vi "Write SC2250 TX Resource Name.vi"(8 "error in (no error)":errorcluster, 10 "SC2250 TX Resource Name":string, 11 "SG SC2250 Path in":refnum<class "SG SC2250 Path.lvclass">) -> (0 "error out":errorcluster, 3 "SG SC2250 Path out":refnum<class "SG SC2250 Path.lvclass">)   [LabVIEW 2023, in "RFFixtureCharact.RFPM.lvlib" / "SG SC2250 Path.lvclass"]
uses:
  SG SC2250 Path.lvclass
  SG SC2250 Path.lvclass/SG SC2250 Path.ctl
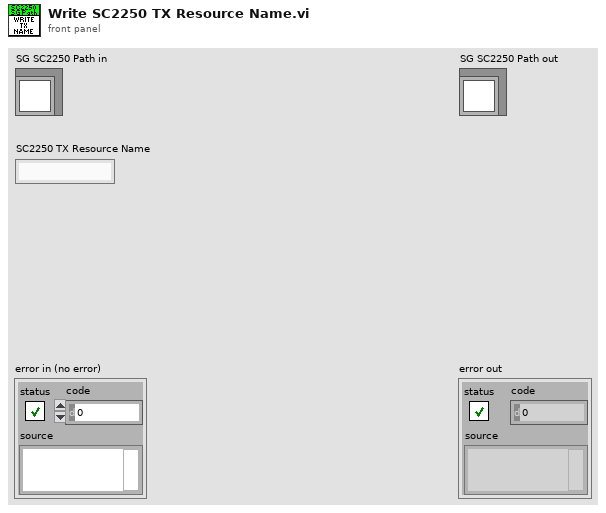
[diagram p1: front panel]
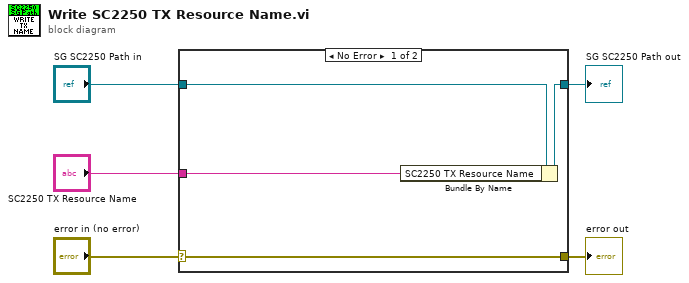
[diagram p0: block diagram]
diagram:
  n1 = case shown="No Error" "error in (no error)" {
    selector: "error in (no error)" -> [w9 w10]
    tunnel: [w9 w10] -> w4
    tunnel: [w7 w11] -> w2
    tunnel: "SG SC2250 Path in" -> [w8 w11]
    tunnel: "SC2250 TX Resource Name" -> [w6 _]
    frame No Error {
      n2 = Bundle By Name(cluster=w8, "SC2250 TX Resource Name"=w6) -> (w7:refnum<class "SG SC2250 Path.lvclass">)
    }
    frame Error {
    }
  }
  "error out" <- w4
  "SG SC2250 Path out" <- w2
